vi "ep_Load Check Error (1 Chan).vi"(7 "additional efficiency information":T1, 8 "error in (no error)":errorcluster, 9 "nameplate information":T2, 10 "speed [RPM]":dbl) -> (0 "error out":errorcluster, 3 "efficiency values [%]":dbl[](array[numeric]))   [LabVIEW 2014, in "NI_EP_Motor Monitoring.lvlib"]
uses:
  <vilib>/addons/Electrical Power/Motor Monitoring/NI_EP_Motor Monitoring.lvlib
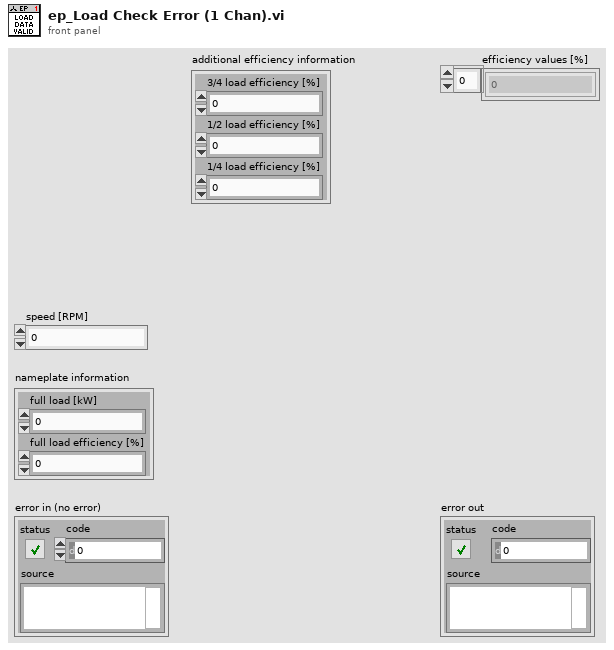
[diagram p1: front panel]
types:
  T1 = cluster{"3/4 load efficiency [%]":dbl, "1/2 load efficiency [%]":dbl, "1/4 load efficiency [%]":dbl}
  T2 = cluster{"full load [kW]":dbl, "full load efficiency [%]":dbl}
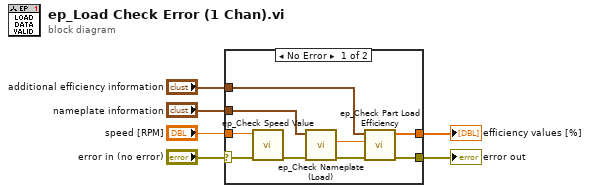
[diagram p0: block diagram]
diagram:
  n1 = case shown="No Error" "error in (no error)" {
    selector: "error in (no error)" -> [w7 w16]
    tunnel: [w14 w16] -> w5
    tunnel: "nameplate information" -> [w9 _]
    tunnel: "speed [RPM]" -> [w15 _]
    tunnel: "additional efficiency information" -> [w13 _]
    tunnel: [w12 _] -> w1
    frame No Error {
      n2 = call <vilib>:"ep_Check Speed Value.vi"("error in (no error)"=w7, "speed [RPM]"=w15) -> ("error out"=w11:errorcluster)  [unwired: 9 in]
      n3 = call <vilib>:"ep_Check Nameplate (Load).vi"("error in (no error)"=w11, "nameplate information"=w9) -> ("error out"=w10:errorcluster, "full load efficiency [%]"=w8:dbl)  [unwired: 8 in]
      n4 = call <vilib>:"ep_Check Part Load Efficiency.vi"("error in (no error)"=w10, "full load efficiency [%]"=w8, "additional efficiency information"=w13) -> ("error out"=w14:errorcluster, "efficiency values [%]"=w12:dbl[])  [unwired: 7 in]
    }
    frame Error {
    }
  }
  "error out" <- w5
  "efficiency values [%]" <- w1
